vi "DiceSubVI.vi"() -> (3 "Numeric":dbl)   [LabVIEW 2018]
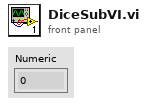
[diagram p1: front panel]
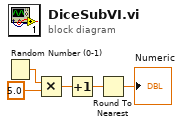
[diagram p0: block diagram]
diagram:
  n1 = Random Number (0-1)() -> (number: 0 to 1=w3:dbl)
  n2 = Multiply(x=w3, y=5.0) -> (x*y=w2:dbl)
  n3 = Increment(x=w2) -> (x+1=w1:dbl)
  n4 = Round To Nearest(number=w1) -> (nearest integer value=→"Numeric":dbl)
